vi "Agilent SNA Read Start and Stop Frequencies.vi"(4 "Passthrough (T)":bool=TRUE, 6 "Channel":i8=1 min=1 max=99 step=1, 7 "Agilent SNA & SWP":T1, 8 "error in (no error)":errorcluster, 11 "VISA Resource Names":T2) -> (0 "error out":errorcluster, 2 "Start/Stop Freqs, MHz":cluster{"Fstart":dbl, "Fstop":dbl}, 3 "dup VISA Resource Names":T2)   [LabVIEW 2011]
doc: "This VI for the HP8753B Network Analyzers reads the stimulus values. Except when performing log sweeps and freq list sweeps, this VI uses the start and stop values and the number of points to calcuate the stimulus values."
uses:
  TypeDefs/Agilent SNA VISA.ctl
  TypeDefs/Agilent SNA Instrument Info.ctl
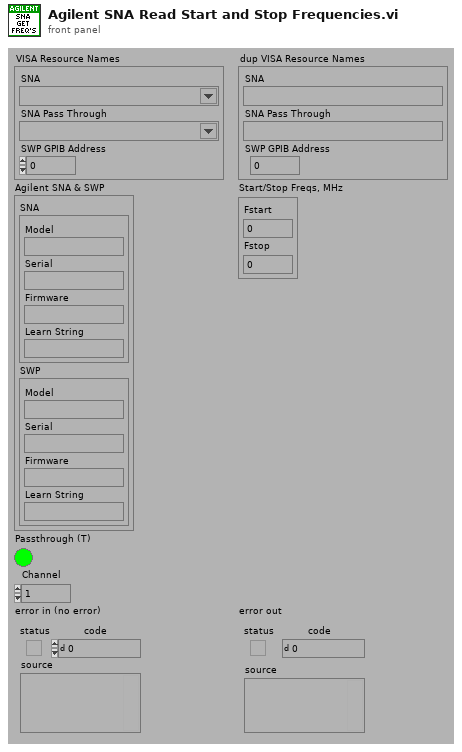
[diagram p1: front panel]
types:
  T1 = typedef "Agilent SNA Instrument Info.ctl" = cluster{"SNA":cluster{"Model":string, "Serial":string, "Firmware":string, "Learn String":string}, "SWP":cluster{"Model":string, "Serial":string, "Firmware":string, "Learn String":string}}
  T2 = typedef "Agilent SNA VISA.ctl" = cluster{"SNA":refnum<visa-resource-name>, "SNA Pass Through":refnum<visa-resource-name>, "SWP GPIB Address":i32}
  T3 = typedef "Agilent SNA Sweep Type.ctl" = enum32{"Linear Sweep", "CW Time Sweep", "Frequency List"}
  T4 = typedef "Agilent SNA Model.ctl" = enum16{"Not Supported", "8757X"}
  T5 = typedef "Agilent SNA SWP Model.ctl" = enum16{"Not Supported", "836XXX", "8375XX", "E82X7D"}
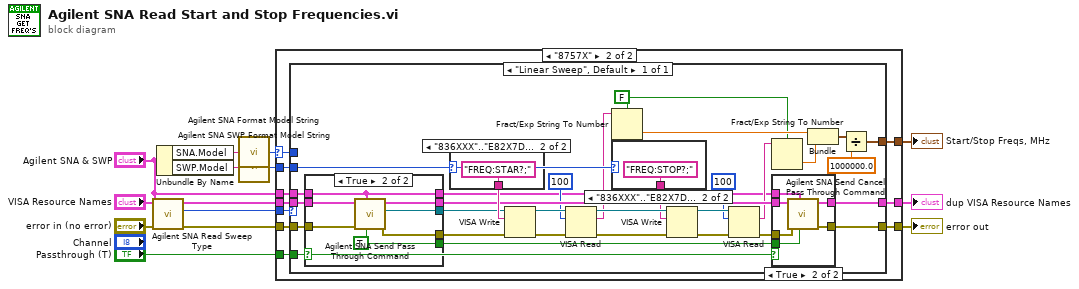
[diagram p0: block diagram]
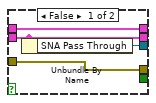
[diagram p4: hidden frame]
diagram:
  n1 = call "Agilent SNA Read Sweep Type.vi"("Agilent SNA & SWP"="Agilent SNA & SWP", "error in (no error)"="error in (no error)", "VISA Resource Names"="VISA Resource Names") -> ("error out"=w10:errorcluster, "Sweep Type"=w12:T3, "dup VISA Resource Names"=w11:T2)  [unwired: 1 in, 5 out]
  n2 = Unbundle By Name("Agilent SNA & SWP") -> ("SNA.Model"=w8:string, "SWP.Model"=w4:string)
  n3 = call "Agilent SNA Format Model String.vi"("Model String"=w8) -> ("Model"=w6:T4)
  n4 = call "Agilent SNA SWP Format Model String.vi"("Model String"=w4) -> ("Model"=w3:T5)
  n5 = case shown="\"8757X\"" w6 {
    selector: w6 -> [_ w20]
    tunnel: [w16 w26] -> w14
    tunnel: w12 -> [_ w25]
    tunnel: w11 -> [w15 w24]
    tunnel: w10 -> [w16 w23]
    tunnel: [_ w22] -> w9
    tunnel: "Agilent SNA & SWP" -> [_ w21]
    tunnel: w3 -> [_ w19]
    tunnel: [w15 w18] -> w2
    tunnel: "Passthrough (T)" -> [_ w17]
    frame "Not Supported" {
    }
    frame "8757X" {
      n6 = case shown="\"Linear Sweep\", Default" w25 {
        tunnel: w24 -> [w53]
        tunnel: w23 -> [w54]
        tunnel: [w47] -> w26
        tunnel: [w49] -> w22
        tunnel: w20 -> [_]
        tunnel: w21 -> [w46]
        tunnel: w19 -> [w36]
        tunnel: [w29] -> w18
        tunnel: w17 -> [w27]
        frame "Linear Sweep", Default {
          w31 = FALSE ("use system decimal point (T)")
          n7 = case shown="True" w27 {
            tunnel: [w67 w76] -> w56
            tunnel: w54 -> [w68 w75]
            tunnel: w53 -> [w66 w74]
            tunnel: [w68 w73] -> w52
            tunnel: w46 -> [w69 w70]
            tunnel: [w66 w72] -> w45
            tunnel: [_ w71] -> w30
            tunnel: [w69 w70] -> w28
            frame False {
              n8 = Unbundle By Name(w66) -> ("SNA Pass Through"=w67:refnum<visa-resource-name>)
            }
            frame True {
              w71 = TRUE ("SCPI? (F)")
              n9 = call "Agilent SNA Send Pass Through Command.vi"("SCPI? (F)"=w71, "Agilent SNA & SWP"=w70, "error in (no error)"=w75, "VISA Resource Names"=w74) -> ("error out"=w73:errorcluster, "SNA Pass Through"=w76:refnum<visa-resource-name>, "dup VISA Resource Names"=w72:T2)  [unwired: 5 out]
            }
          }
          n10 = case shown="\"836XXX\"..\"E82X7D\"" w36 {
            tunnel: [_ "FREQ:STAR?;" ("format string")] -> w57
            frame "Not Supported" {
            }
            frame "836XXX".."E82X7D" {
            }
          }
          n11 = VISA Write(VISA resource name=w56, write buffer=w57, error in (no error)=w52) -> (VISA resource name out=w55:refnum<visa-resource-name>, error out=w51:errorcluster)  [unwired: 1 out]
          n12 = VISA Read(VISA resource name=w55, byte count=u32 100, error in (no error)=w51) -> (VISA resource name out=w42:refnum<visa-resource-name>, read buffer=w35:string, error out=w43:errorcluster)  [unwired: 1 out]
          n13 = Fract/Exp String To Number(use system decimal point (T)=w31, string=w35) -> (number=w34:dbl)  [unwired: 3 out]
          n14 = case shown="\"836XXX\"..\"E82X7D\"" w36 {
            tunnel: [_ "FREQ:STOP?;" ("format string")] -> w37
            frame "Not Supported" {
            }
            frame "836XXX".."E82X7D" {
            }
          }
          n15 = VISA Write(VISA resource name=w42, write buffer=w37, error in (no error)=w43) -> (VISA resource name out=w41:refnum<visa-resource-name>, error out=w44:errorcluster)  [unwired: 1 out]
          n16 = VISA Read(VISA resource name=w41, byte count=u32 100, error in (no error)=w44) -> (read buffer=w33:string, error out=w40:errorcluster)  [unwired: 2 out]
          n17 = Fract/Exp String To Number(use system decimal point (T)=w31, string=w33) -> (number=w32:dbl)  [unwired: 3 out]
          n18 = case shown="True" w27 {
            tunnel: [w59 w65] -> w47
            tunnel: w45 -> [w58 w64]
            tunnel: w40 -> [w59 w63]
            tunnel: w30 -> [_ w62]
            tunnel: [w58 w61] -> w29
            tunnel: w28 -> [_ w60]
            frame False {
            }
            frame True {
              n19 = call "Agilent SNA Send Cancel Pass Through Command.vi"("SCPI? (F)"=w62, "Agilent SNA & SWP"=w60, "error in (no error)"=w63, "VISA Resource Names"=w64) -> ("error out"=w65:errorcluster, "dup VISA Resource Names"=w61:T2)  [unwired: 6 out]
            }
          }
          n20 = Bundle(w34, w32) -> (w50:cluster{dbl, dbl})  [unwired: 1 out]
          n21 = Divide(x=w50, y=1000000.0 ("x")) -> (x/y=w49:cluster{dbl, dbl})
        }
      }
    }
  }
  "dup VISA Resource Names" <- w2
  "error out" <- w14
  "Start/Stop Freqs, MHz" <- w9
